vi "task 1.vi"() -> ()   [LabVIEW 2020]
panel:
  in  "Tab Control":enum32{"Page 1", "Page 2"}(tab)
  in  "log":bool
  in  "Username":string
  in  "Password":string
  out "?":bool
  out "?":bool
  in  "read":bool
  in  "Home Button":bool
  in  "stop":bool
  in  "Path":path
  out "text":string
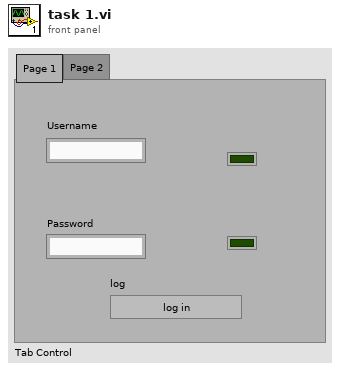
[diagram p1: front panel]
types:
  T1 = enum16{"open", "replace", "create", "open or create", "replace or create", "replace or create with confirmation"}
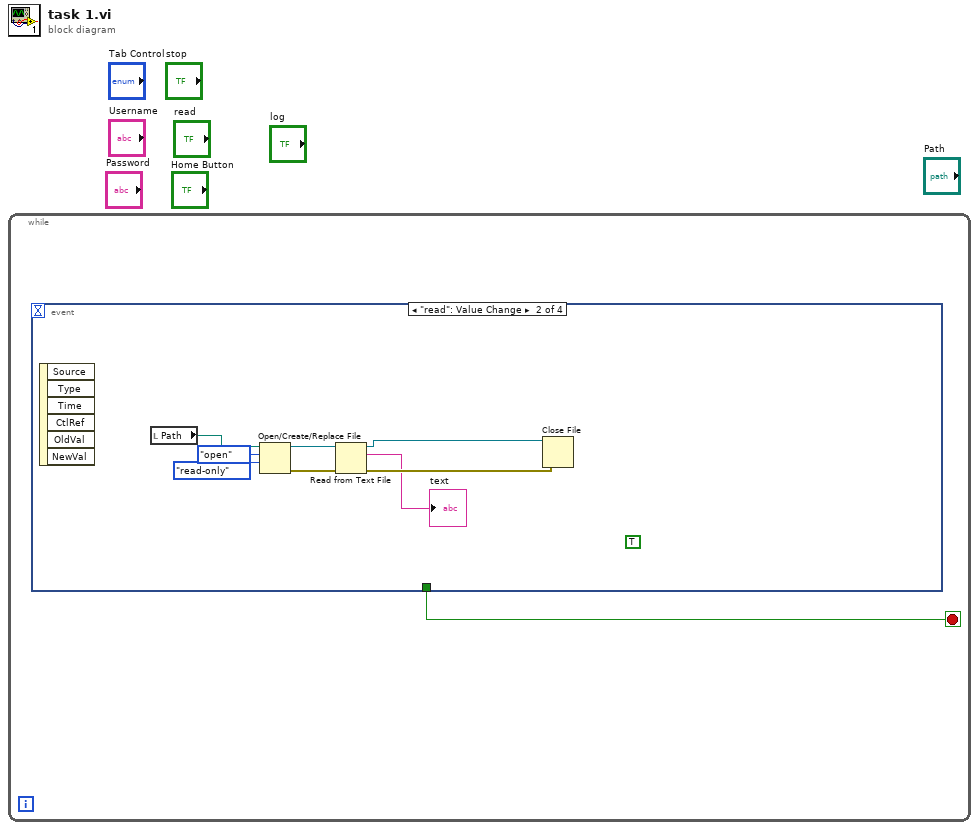
[diagram p0: block diagram]
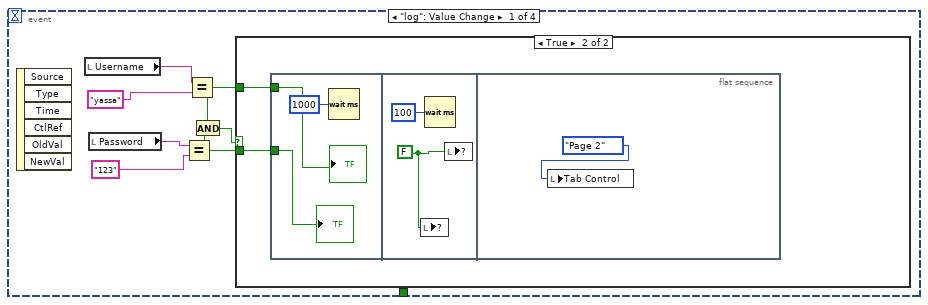
[diagram p2: hidden frame]
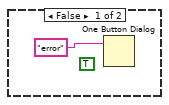
[diagram p3: hidden frame]
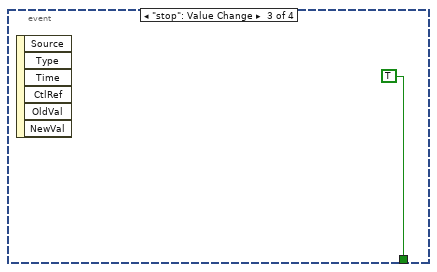
[diagram p4: hidden frame]
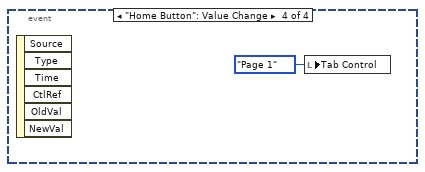
[diagram p5: hidden frame]
diagram:
  n1 = while {
    stop <- w1 stop-if-true
    (unwired) TRUE
    n2 = event shown="[1] \"read\": Value Change" {
      selector: _ -> [_ _ _ _]
      dyn-events: _ -> [_ _ _ _]
      timeout: _ -> [_ _ _ _]
      tunnel: [_ _ TRUE _] -> w1
      event "log": Value Change {
        n3 = event-data() -> ()  [unwired: 1 in, 6 out]
        n4 = local read "Username"() -> (w5:string)
        n5 = local read "Password"() -> (w6:string)
        n6 = Equal?(x=w6, y="123") -> (x = y?=w2:bool)
        n7 = Equal?(x=w5, y="yassa") -> (x = y?=w3:bool)
        n8 = And(x=w3, y=w2) -> (x .and. y?=w4:bool)
        n9 = case shown="True" w4 {
          tunnel: w3 -> [_ w11]
          tunnel: w2 -> [_ w10]
          frame False {
            (unwired) TRUE ("true")
            n10 = One Button Dialog(message="error") -> ()  [unwired: 1 in, 1 out]
          }
          frame True {
            n11 = flat-sequence {
              tunnel: w11 -> [w13]
              tunnel: w10 -> [w12]
              frame #0 {
                n12 = Wait (ms)(milliseconds to wait=u32 1000) -> ()  [unwired: 1 out]
                "?" <- w13
                "?" <- w12
              }
              frame #1 {
                w16 = FALSE
                n13 = local write item#9(w16) -> ()
                n14 = Wait (ms)(milliseconds to wait=u32 100) -> ()  [unwired: 1 out]
                n15 = local write item#10(w16) -> ()
              }
              frame #2 {
                n16 = local write "Tab Control"(enum32{"Page 1", "Page 2"}."Page 2" ("Tab Control")) -> ()
              }
            }
          }
        }
      }
      event "read": Value Change {
        n17 = event-data() -> ()  [unwired: 1 in, 6 out]
        n18 = local read "Path"() -> (w25:path)
        n19 = Open/Create/Replace File(file path (use dialog)=w25, operation (0:open)=T1."open", access (0:read/write)=enum16{"read/write", "read-only", "write-only"}."read-only") -> (refnum out=w22:refnum<file>, error out=w23:errorcluster)  [unwired: 3 in, 1 out]
        n20 = Read from Text File(file (use dialog)=w22, error in=w23) -> (refnum out=w21:refnum<file>, text=→"text":string, error out=w24:errorcluster)  [unwired: 2 in, 1 out]
        n21 = Close File(refnum=w21, error in=w24) -> ()  [unwired: 2 out]
      }
      event "stop": Value Change {
        n22 = event-data() -> ()  [unwired: 1 in, 6 out]
      }
      event "Home Button": Value Change {
        n23 = event-data() -> ()  [unwired: 1 in, 6 out]
        n24 = local write "Tab Control"(enum32{"Page 1", "Page 2"}."Page 1" ("Tab Control")) -> ()
      }
    }
  }
